vi "Write Function Definition.vi"(8 "error in":errorcluster, 10 "master function definition":refnum<class "Master Function Definition.lvclass">, 11 "Modbus master in":refnum<class "Modbus Master.lvclass">) -> (0 "error out":errorcluster, 3 "Modbus master out":refnum<class "Modbus Master.lvclass">)   [LabVIEW 2012, in "Modbus Master.lvclass"]
doc: "This VI is an accessor for the function definition stored in the Modbus master instance. This accessor can be used as a property node. This function definition is used by the master to determine how to pack and unpack Modbus protocol data units."
uses:
  Modbus Master.lvclass
  Master Function Definition/Master Function Definition.lvclass
  Modbus Master.lvclass/Modbus Master.ctl
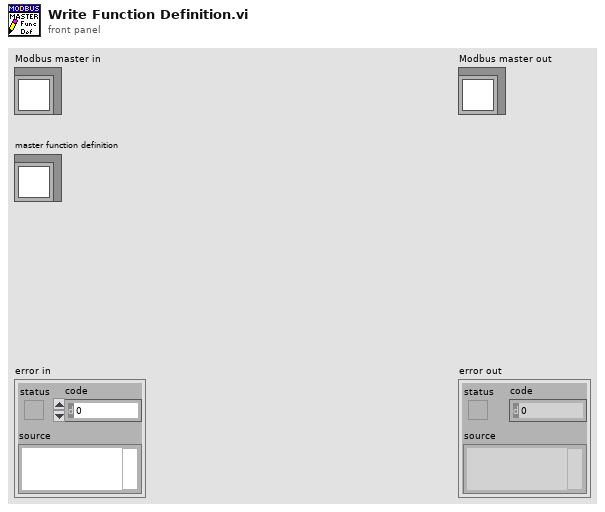
[diagram p1: front panel]
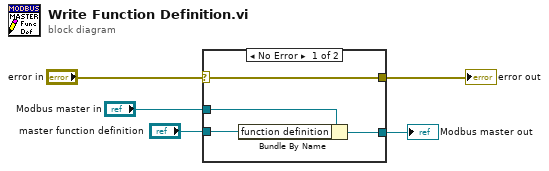
[diagram p0: block diagram]
diagram:
  n1 = case shown="No Error" "error in" {
    selector: "error in" -> [w9 w10]
    tunnel: [w9 w10] -> w4
    tunnel: [w7 w11] -> w2
    tunnel: "Modbus master in" -> [w8 w11]
    tunnel: "master function definition" -> [w6 _]
    frame No Error {
      n2 = Bundle By Name(cluster=w8, "function definition"=w6) -> (w7:refnum<class "Modbus Master.lvclass">)
    }
    frame Error {
    }
  }
  "error out" <- w4
  "Modbus master out" <- w2
